vi "ErrorDialog.vi"(1 "error in":errorcluster, 2 "message":string="Failed!\nDetail:\n") -> ()   [LabVIEW 2015]
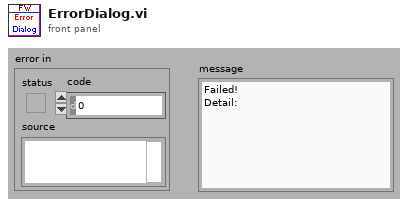
[diagram p1: front panel]
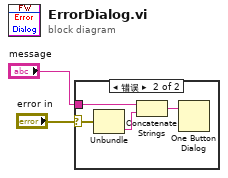
[diagram p0: block diagram]
diagram:
  n1 = case shown="错误" "error in" {
    selector: "error in" -> [_ w6]
    tunnel: "message" -> [_ w3]
    frame No Error {
    }
    frame Error {
      n2 = Unbundle(w6) -> ("source"=w5:string)  [unwired: 2 out]
      n3 = Concatenate Strings(w3, w5) -> (w4:string)
      n4 = One Button Dialog(message=w4) -> ()  [unwired: 1 in, 1 out]
    }
  }
